vi "Button Appearance Properties.vi"(8 "Error In":errorcluster, 9 "Bool Refnum":refnum<vi>, 11 "Display State In":T1 caption="State") -> (0 "Error Out":errorcluster, 3 "Display State Out":T1 caption="State", 4 "Change":bool)   [LabVIEW 2012, in "Hover Button.xctl"]
doc: "This vi is the interactive property page used to define the color and text properties of the Hover Button."
uses:
  Hover Button.xctl
  State.ctl
  Button Colors.ctl
  Font Properties.ctl
  Color Select.ctl
  <vilib>/Utility/miscctls.llb/LVBoundsTypeDef.ctl
panel:
  in  "Tab Control":enum32{"Appearance", "Font"}(tab)
  in  "On":u32(colorbox)=16860
  in  "Text Color":u32(colorbox)=16448250
  in  "Hover On":u32(colorbox)=16776960
  in  "Hover Text Color":u32(colorbox)
  in  "Example Button":bool
  in  "On text":string
  in  "Off Text":string="Off"
  in  "Off":u32(colorbox)=16860
  in  "Hover Off":u32(colorbox)=16776960
  in  "Show Boolean Text":bool
  in  "Mulitiple strings":bool
  in  "Size":u32=1 min=1 step=1
  in  "Strikeout":bool
  in  "Underline":bool
  in  "Italic":bool
  in  "Bold":bool
  in  "Plain":bool
  out "Example String":string="The quick brown fox jumped over the lazy dog"
  in  "Font":u16(ring) items=["App Font", "Sys Font", "Dlg Font", "ADMUI3.fon", "Agency FB", "Agency FB Bold", "Arial", "Arial Baltic", "Arial Black", "Arial Bold", "Arial Bold Italic", "Arial CE", "Arial CYR", "Arial Greek", "Arial Italic", "Arial Narrow", "Arial Narrow Bold", "Arial Narrow Bold Italic", "Arial Narrow Italic", "Arial Rounded MT Bold", "Arial TUR", "Arial Unicode MS", "Blackadder ITC", "Bodoni MT", "Bodoni MT Black", "Bodoni MT Black Italic", "Bodoni MT Bold", "Bodoni MT Bold Italic", "Bodoni MT Condensed", "Bodoni MT Condensed Bold", "Bodoni MT Condensed Bold Italic", "Bodoni MT Condensed Italic", "Bodoni MT Italic", "Book Antiqua", "Book Antiqua Bold", "Book Antiqua Bold Italic", "Book Antiqua Italic", "Bookman Old Style", "Bookman Old Style Bold", "Bookman Old Style Bold Italic", "Bookman Old Style Italic", "Bookshelf Symbol 7", "Bradley Hand ITC", "Calibri", "Calibri Bold", "Calibri Bold Italic", "Calibri Italic", "Calisto MT", "Calisto MT Bold", "Calisto MT Bold Italic", "Calisto MT Italic", "Cambria & Cambria Math", "Cambria Bold", "Cambria Bold Italic", "Cambria Italic", "Candara", "Candara Bold", "Candara Bold Italic", "Candara Italic", "Castellar", "Century Gothic", "Century Gothic Bold", "Century Gothic Bold Italic", "Century Gothic Italic", "Century Schoolbook", "Century Schoolbook Bold", "Century Schoolbook Bold Italic", "Century Schoolbook Italic", "Comic Sans MS", "Comic Sans MS Bold", "Consolas", "Consolas Bold", "Consolas Bold Italic", "Consolas Italic", "Constantia", "Constantia Bold", "Constantia Bold Italic", "Constantia Italic", "Copperplate Gothic Bold", "Copperplate Gothic Light", "Corbel", "Corbel Bold", "Corbel Bold Italic", "Corbel Italic", "Courier 10,12,15", "Courier New", "Courier New Baltic", "Courier New Bold", "Courier New Bold Italic", "Courier New CE", "Courier New CYR", "Courier New Greek", "Courier New Italic", "Courier New TUR", "Curlz MT", "Edwardian Script ITC", "Elephant", "Elephant Italic", "Engravers MT", "Eras Bold ITC", "Eras Demi ITC", "Eras Light ITC", "Eras Medium ITC", "Estrangelo Edessa", "Estrangelo Edessa", "Euro Sign", "Felix Titling", "Forte", "Franklin Gothic Book", "Franklin Gothic Book Italic", "Franklin Gothic Demi", "Franklin Gothic Demi Cond", "Franklin Gothic Demi Italic", "Franklin Gothic Heavy", "Franklin Gothic Heavy Italic", "Franklin Gothic Medium", "Franklin Gothic Medium Cond", "Franklin Gothic Medium Italic", "French Script MT", "Garamond", "Garamond Bold", "Garamond Italic", "Gautami", "Georgia", "Georgia Bold", "Georgia Bold Italic", "Georgia Italic", "Gigi", "Gill Sans MT", "Gill Sans MT Bold", "Gill Sans MT Bold Italic", "Gill Sans MT Condensed", "Gill Sans MT Ext Condensed Bold", "Gill Sans MT Italic", "Gill Sans Ultra Bold", "Gill Sans Ultra Bold Condensed", "Gloucester MT Extra Condensed", "Goudy Old Style", "Goudy Old Style Bold", "Goudy Old Style Italic", "Goudy Stout", "HE_TERMINAL", "Haettenschweiler", "Helv", "Helvetica", "Impact", "Imprint MT Shadow", "Latha", "Lucida Console", "Lucida Sans Demibold Italic", "Lucida Sans Demibold Roman", "Lucida Sans Italic", "Lucida Sans Regular", "Lucida Sans Typewriter Bold", "Lucida Sans Typewriter Bold Oblique", "Lucida Sans Typewriter Oblique", "Lucida Sans Typewriter Regular", "Lucida Sans Unicode", "MS Outlook", "MS Reference Sans Serif", "MS Reference Specialty", "MS Sans Serif 8,10,12,14,18,24", "MS Serif 8,10,12,14,18,24", "MS Shell Dlg", "MS Shell Dlg 2", "MT Extra", "Maiandra GD", "Mangal", "Microsoft Sans Serif", "Modern", "Monotype Corsiva", "Mv Boli", "OCR A Extended", "Palace Script MT", "Palatino Linotype", "Palatino Linotype Bold", "Palatino Linotype Bold Italic", "Palatino Linotype Italic", "Papyrus", "Perpetua", "Perpetua Bold", "Perpetua Bold Italic", "Perpetua Italic", "Perpetua Titling MT Bold", "Perpetua Titling MT Light", "Pristina", "Raavi", "Rage Italic", "Rockwell", "Rockwell Bold", "Rockwell Bold Italic", "Rockwell Condensed", "Rockwell Condensed Bold", "Rockwell Extra Bold", "Rockwell Italic", "Roman", "Script", "Script MT Bold", "Shruti", "Small Fonts", "Sylfaen", "Symbol", "Symbol 8,10,12,14,18,24", "Tahoma", "Tahoma Bold", "Times", "Times New Roman", "Times New Roman Baltic", "Times New Roman Bold", "Times New Roman Bold Italic", "Times New Roman CE", "Times New Roman CYR", "Times New Roman Greek", "Times New Roman Italic", "Times New Roman TUR", "Tms Rmn", "Trebuchet MS", "Trebuchet MS Bold", "Trebuchet MS Bold Italic", "Trebuchet MS Italic", "Tunga", "Tw Cen MT", "Tw Cen MT Bold", "Tw Cen MT Bold Italic", "Tw Cen MT Condensed", "Tw Cen MT Condensed Bold", "Tw Cen MT Condensed Extra Bold", "Tw Cen MT Italic", "Verdana", "Verdana Bold", "Verdana Bold Italic", "Verdana Italic", "WST_Czec", "WST_Engl", "WST_Fren", "WST_Germ", "WST_Ital", "WST_Span", "WST_Swed", "Webdings", "WingDings", "Wingdings 2", "Wingdings 3", "ZWAdobeF"]
  in  "Alignment":enum16{"Left", "Center", "Right"}(ring)
  in  "Cancel Button":bool
  in  "OK Button":bool
  # "Appearance"
  # "Colors"
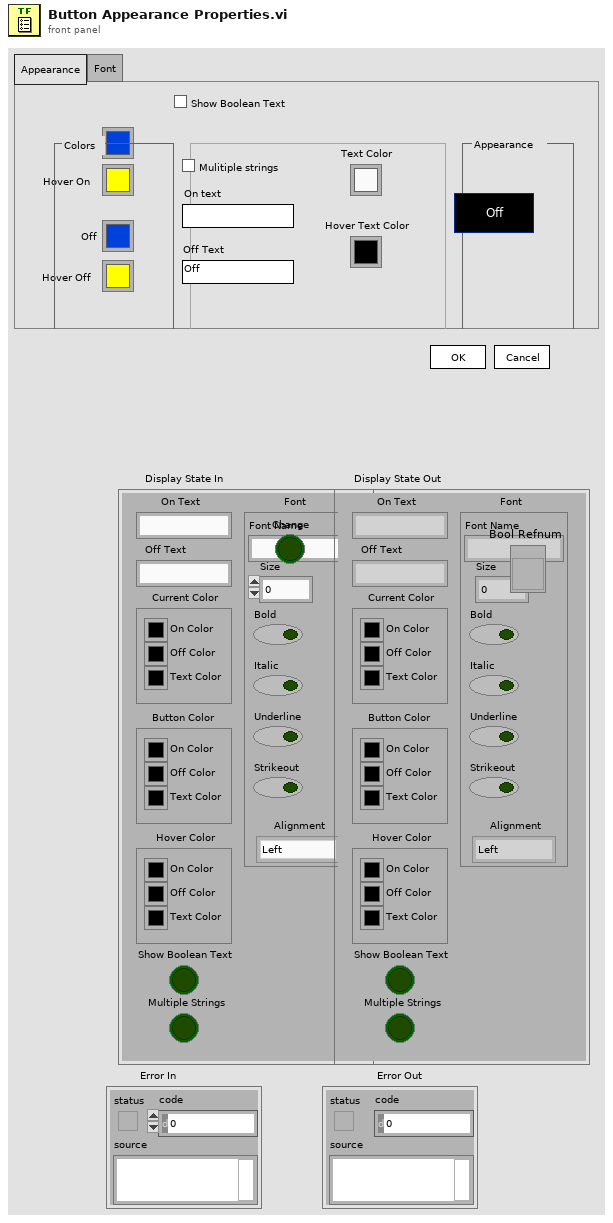
[diagram p1: front panel]
types:
  T1 = typedef "Hover Button.xctl/State.ctl" = cluster{"On Text":string, "Off Text":string, "Current Color":T2, "Button Color":T2, "Hover Color":T2, "Show Boolean Text":bool, "Multiple Strings":bool, "Font":T3}
  T2 = typedef "Hover Button.xctl/Button Colors.ctl" = cluster{"On Color":u32, "Text Color":u32, "Off Color":u32}
  T3 = typedef "Hover Button.xctl/Font Properties.ctl" = cluster{"Font Name":string, "Size":u32, "Bold":bool, "Italic":bool, "Underline":bool, "Strikeout":bool, "Alignment":enum16{"Left", "Center", "Right"}}
  T4 = typedef "Hover Button.xctl/Color Select.ctl" = enum16{"Current Color", "Button Color", "Hover Color"}
  T5 = typedef "LVBoundsTypeDef.ctl" = cluster{"Width":u32, "Height":u32}
  T6 = cluster{"Text Color":u32, "Background Color":u32}
  T7 = typedef "LVPositionTypeDef.ctl" = cluster{"Left":i32, "Top":i32}
  T8 = cluster{"On Text":bool, "Off Text":bool, "Current Color":cluster{"On Color":bool, "Text Color":bool, "Off Color":bool}, "Button Color":cluster{"On Color":bool, "Text Color":bool, "Off Color":bool}, "Hover Color":cluster{"On Color":bool, "Text Color":bool, "Off Color":bool}, "Show Boolean Text":bool, "Multiple Strings":bool, "Font":cluster{"Font Name":bool, "Size":bool, "Bold":bool, "Italic":bool, "Underline":bool, "Strikeout":bool, "Alignment":bool}}
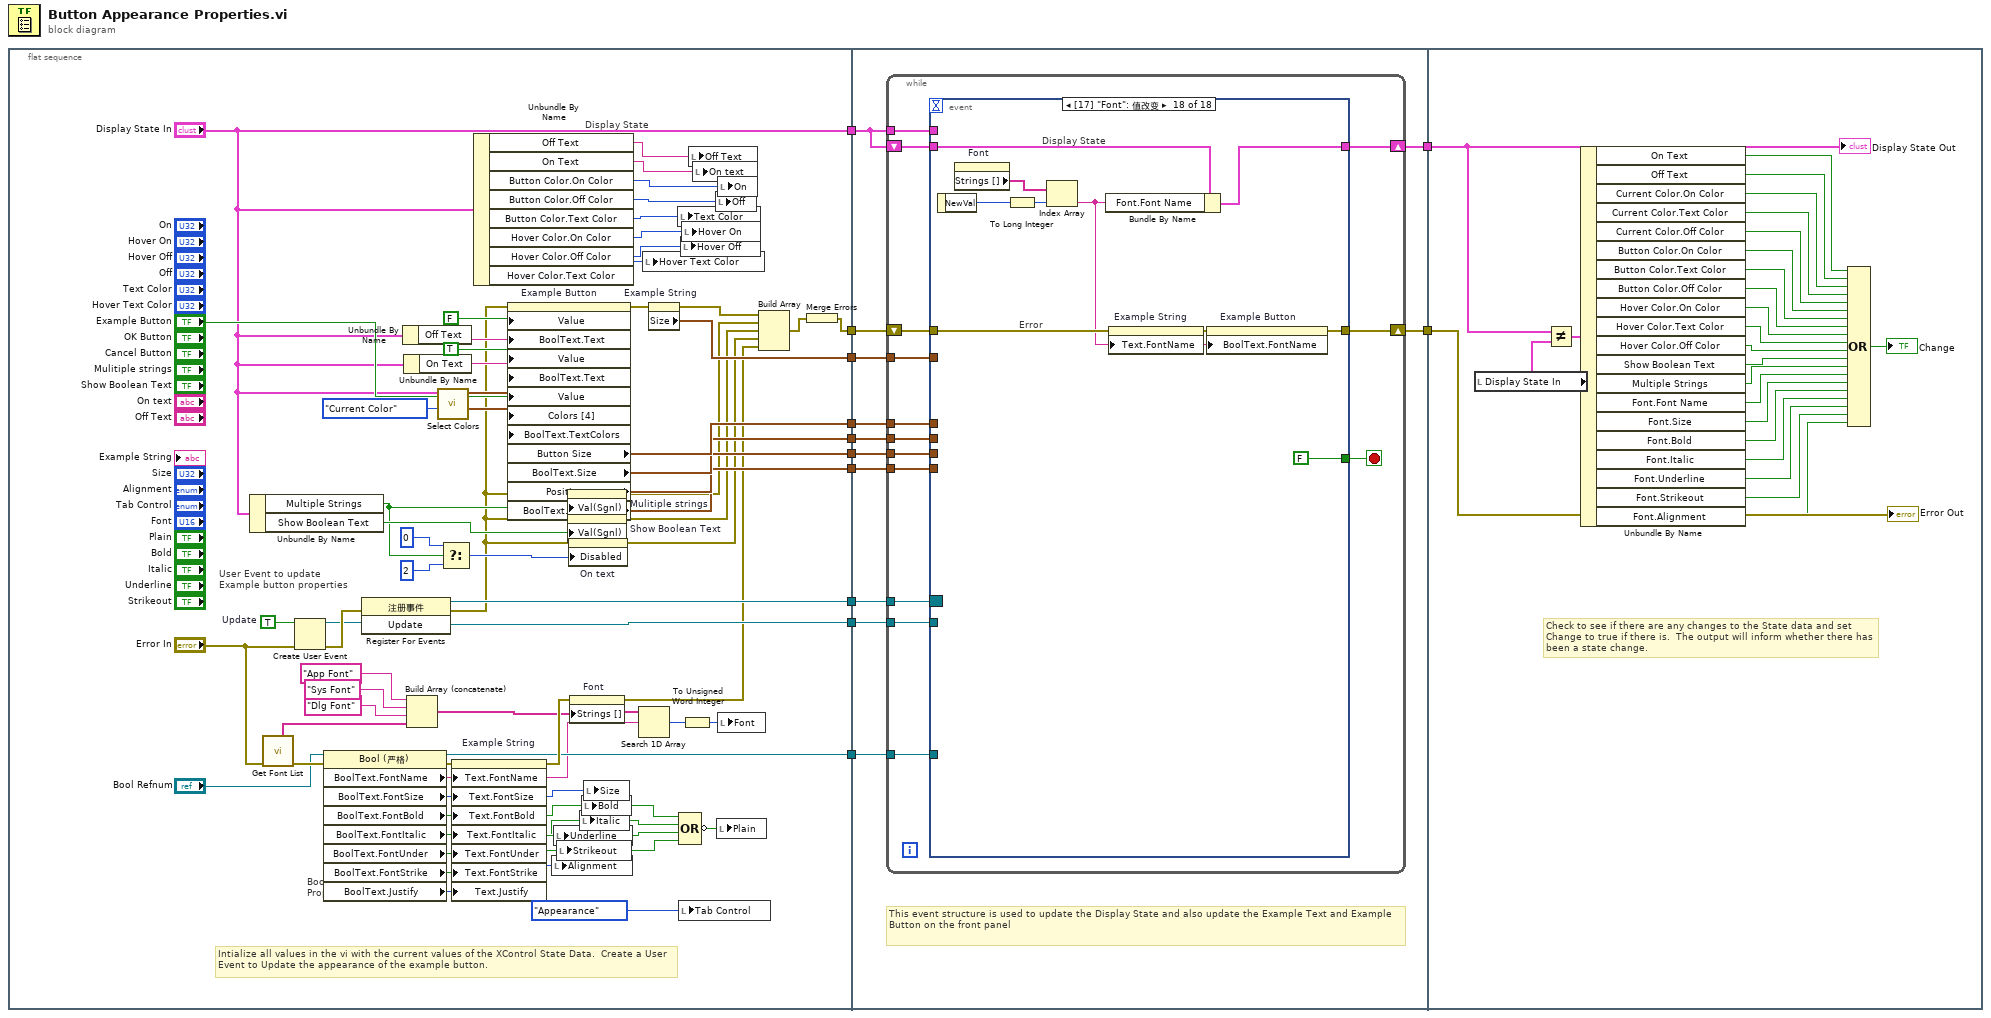
[diagram p0: block diagram]
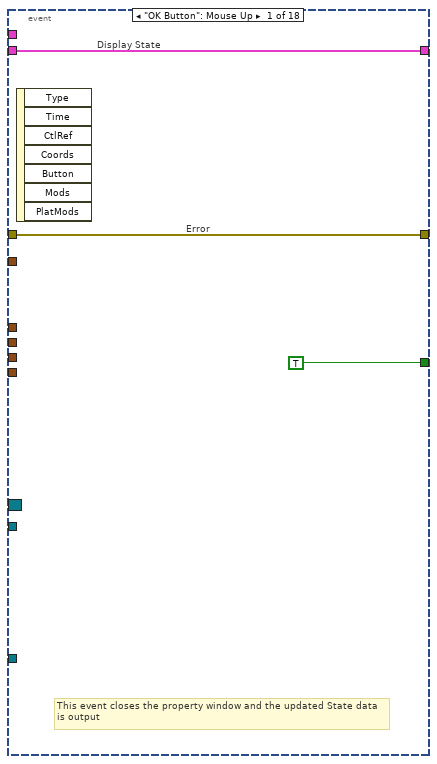
[diagram p2: hidden frame]
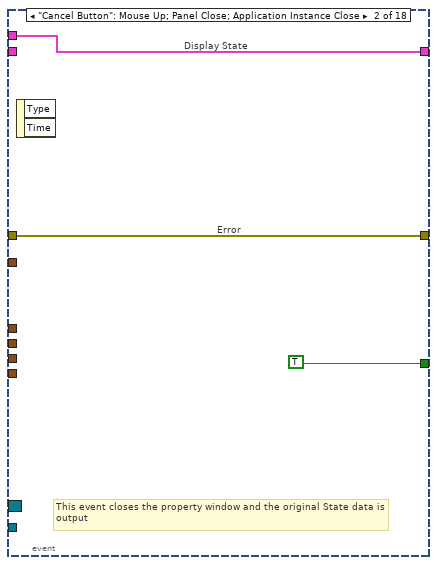
[diagram p3: hidden frame]
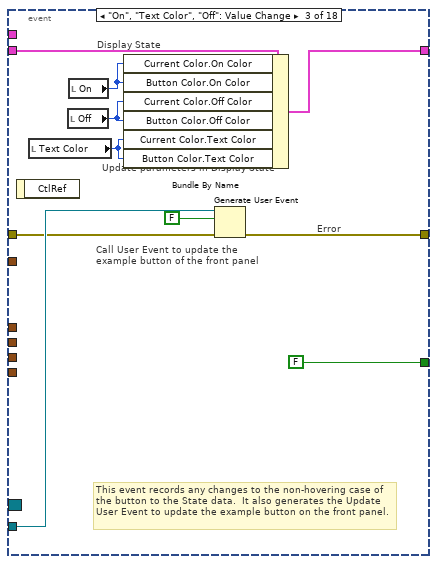
[diagram p4: hidden frame]
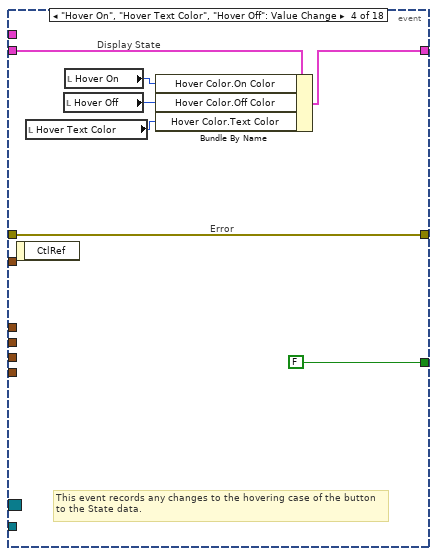
[diagram p5: hidden frame]
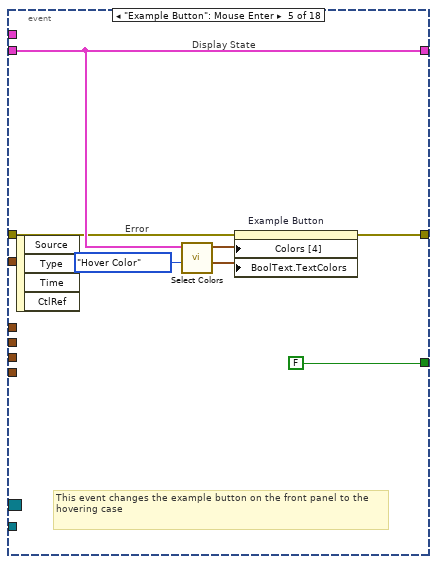
[diagram p6: hidden frame]
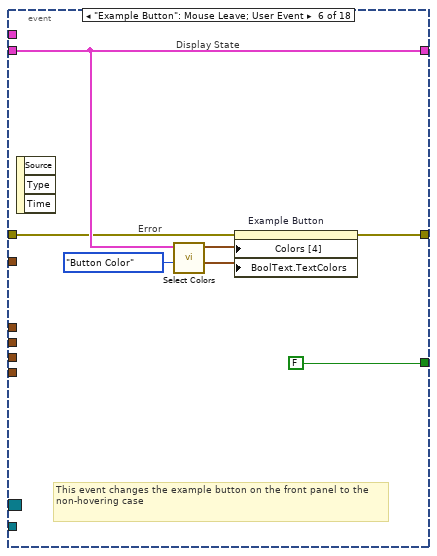
[diagram p7: hidden frame]
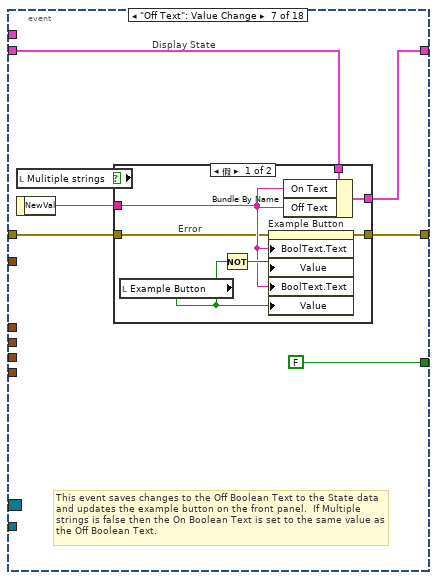
[diagram p8: hidden frame]
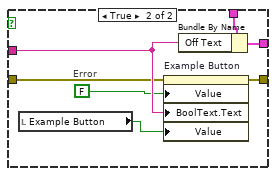
[diagram p9: hidden frame]
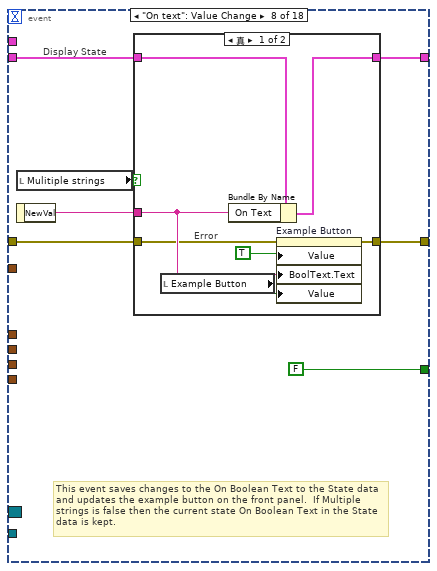
[diagram p10: hidden frame]
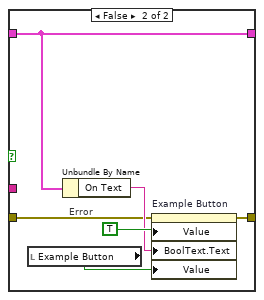
[diagram p11: hidden frame]
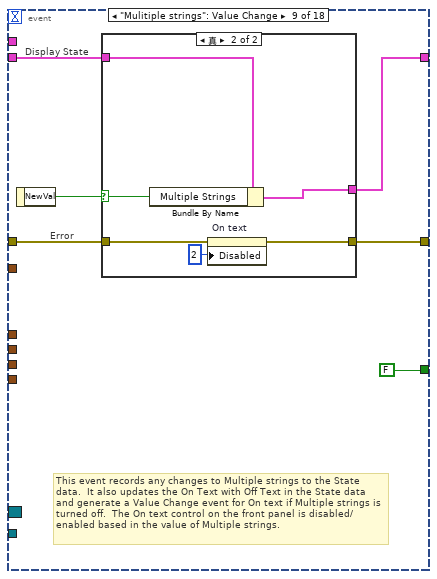
[diagram p12: hidden frame]
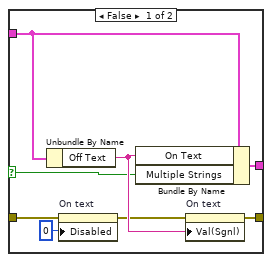
[diagram p13: hidden frame]
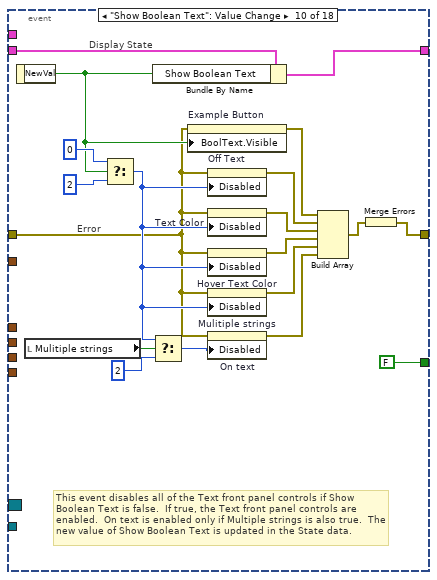
[diagram p14: hidden frame]
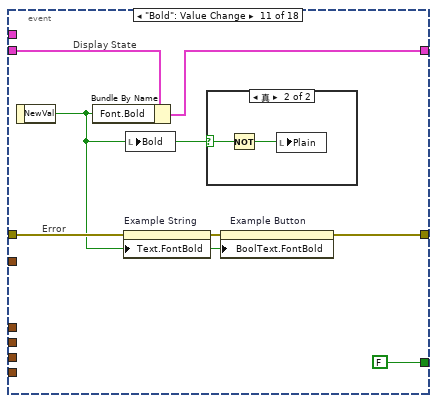
[diagram p15: hidden frame]
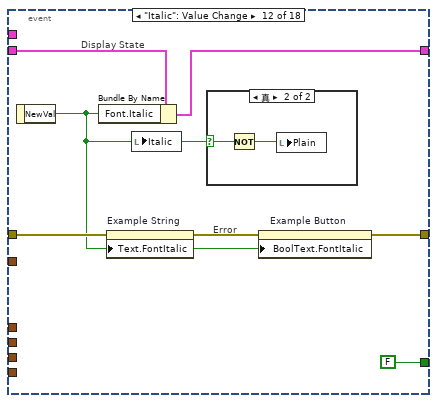
[diagram p17: hidden frame]
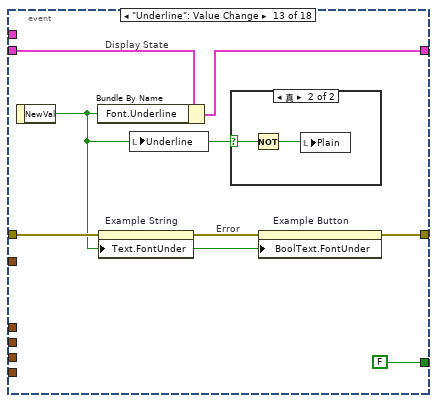
[diagram p19: hidden frame]
diagram:
  n1 = flat-sequence {
    tunnel: ["Display State In"] -> w12
    tunnel: [w26] -> w10
    tunnel: [w25] -> w9
    tunnel: [w54] -> w8
    tunnel: [w47] -> w6
    tunnel: [w27] -> w5
    tunnel: [w33] -> w4
    tunnel: [w32] -> w3
    tunnel: [w31] -> w2
    tunnel: [w30] -> w1
    tunnel: w12 -> [w86]
    tunnel: [w85] -> w11
    tunnel: w10 -> [w84]
    tunnel: w9 -> [w83]
    tunnel: w8 -> [w82]
    tunnel: [w81] -> w7
    tunnel: w6 -> [w80]
    tunnel: w5 -> [w79]
    tunnel: w4 -> [w78]
    tunnel: w3 -> [w77]
    tunnel: w2 -> [w76]
    tunnel: w1 -> [w75]
    tunnel: w11 -> [w317]
    tunnel: w7 -> [w302]
    frame #0 {
      w72 = TRUE  # Update
      # "User Event to update\nExample button properties"
      # "Boolean Button Reference\nProperties"
      # "Display State"
      # "Intialize all values in the vi with the current values of the XControl State Data.  Create a User Event to Update the appearance of the example button."
      n2 = Unbundle By Name("Display State In") -> ("Multiple Strings"=w55:bool, "Show Boolean Text"=w58:bool)
      n3 = call "Get Font List.vi"("Error In"="Error In") -> ("Error Out"=w74:errorcluster, "Font Array"=w28:string[])  [unwired: 9 in]
      n4 = Create User Event(user event datatype=w72, error in="Error In") -> (user event=w25:refnum<user-event>, error out=w35:errorcluster)
      n5 = property class="Bool (严格)"(reference="Bool Refnum", error in=w74) -> (reference out=w47:refnum<vi>, error out=w36:errorcluster, "BoolText.FontName"=w37:string, "BoolText.FontSize"=w38:u32, "BoolText.FontBold"=w39:bool, "BoolText.FontItalic"=w40:bool, "BoolText.FontUnder"=w41:bool, "BoolText.FontStrike"=w42:bool, "BoolText.Justify"=w43:enum16{"Left", "Center", "Right"})
      n6 = register-events(error in=w35, w25) -> (reference out=w26:refnum<event-registration>, error out=w19:errorcluster)  [unwired: 1 in]
      n7 = Unbundle By Name("Display State In") -> ("Off Text"=w67:string)
      n8 = Unbundle By Name("Display State In") -> ("On Text"=w66:string)
      n9 = Build Array (concatenate)("App Font", "Sys Font", "Dlg Font", w28) -> (w50:string[])
      n10 = call "Select Colors.vi"("Color Select"=Color_Select."Current Color", "State"="Display State In") -> ("Text Colors"=w56:T6, "Button Colors"=w57:cluster{"FG":u32, "BG":u32}[])  [unwired: 8 in]
      n11 = Select(t=u8 0, s=w55, f=u8 2) -> (s? t:f=w59:u8)
      n12 = property on="Example String" class="Str"(error in=w36, "Text.FontName"=w37, "Text.FontSize"=w38, "Text.FontBold"=w39, "Text.FontItalic"=w40, "Text.FontUnder"=w41, "Text.FontStrike"=w42, "Text.Justify"=w43) -> (error out=w73:errorcluster)  [unwired: 1 in, 1 out]
      n13 = Unbundle By Name("Display State In") -> ("Off Text"=w20:string, "On Text"=w21:string, "Button Color.On Color"=w22:u32, "Button Color.Off Color"=w23:u32, "Button Color.Text Color"=w24:u32, "Hover Color.On Color"=w70:u32, "Hover Color.Off Color"=w69:u32, "Hover Color.Text Color"=w68:u32)
      n14 = property on="Example Button" class="Bool (严格)"(error in=w19, "Value"=FALSE ("Boolean"), "BoolText.Text"=w67, "Value"=TRUE ("Boolean"), "BoolText.Text"=w66, "Value"="Example Button", "Colors [4]"=w57, "BoolText.TextColors"=w56) -> (error out=w29:errorcluster, "Button Size"=w33:T5, "BoolText.Size"=w32:T5, "Position"=w31:T7, "BoolText.Position"=w30:T7)  [unwired: 1 in, 1 out]
      n15 = local write "Alignment"(w43) -> ()
      n16 = local write "Underline"(w41) -> ()
      n17 = local write "Strikeout"(w42) -> ()
      n18 = property on="Mulitiple strings" class="Bool (严格)"(error in=w19, "Val(Sgnl)"=w55) -> (error out=w15:errorcluster)  [unwired: 1 in, 1 out]
      n19 = property on="Show Boolean Text" class="Bool (严格)"(error in=w19, "Val(Sgnl)"=w58) -> (error out=w16:errorcluster)  [unwired: 1 in, 1 out]
      n20 = property on="On text" class="Str"(error in=w19, "Disabled"=w59) -> (error out=w17:errorcluster)  [unwired: 1 in, 1 out]
      n21 = property on="Font" class="Ring (严格)"(error in=w73, "Strings []"=w50) -> (error out=w18:errorcluster)  [unwired: 1 in, 1 out]
      n22 = local write "Italic"(w40) -> ()
      n23 = local write "Bold"(w39) -> ()
      n24 = local write "Size"(w38) -> ()
      n25 = Search 1D Array(1D array=w50, element=w37) -> (index of element=w48:i32)  [unwired: 1 in]
      n26 = local write "Hover Text Color"(w68) -> ()
      n27 = property on="Example String" class="Str"(error in=w29) -> (error out=w14:errorcluster, "Size"=w27:T5)  [unwired: 1 in, 1 out]
      n28 = local write "Text Color"(w24) -> ()
      n29 = Compound Arithmetic op=OR(w39, w40, w41, w42) -> (invert w45:bool)
      n30 = local write "Tab Control"(enum32{"Appearance", "Font"}."Appearance" ("Tab Control")) -> ()
      n31 = local write "Hover Off"(w69) -> ()
      n32 = local write "Hover On"(w70) -> ()
      n33 = To Unsigned Word Integer(number=w48) -> (unsigned 16bit integer=w46:u16)
      n34 = local write "Off Text"(w20) -> ()
      n35 = local write "On text"(w21) -> ()
      n36 = local write "Off"(w23) -> ()
      n37 = local write "Plain"(w45) -> ()
      n38 = local write "On"(w22) -> ()
      n39 = local write "Font"(w46) -> ()
      n40 = Build Array(w14, w15, w16, w17, w18) -> (w13:errorcluster[])
      n41 = Merge Errors(w13) -> (w54:errorcluster)
    }
    frame #1 {
      # "This event structure is used to update the Display State and also update the Example Text and Example Button on the front panel"
      n42 = while {
        tunnel: w86 -> [w97]
        shift-right: [w98] -> w85
        shift-left: w86 -> [w99]
        tunnel: w84 -> [w96]
        tunnel: w83 -> [w95]
        shift-right: [w93] -> w81
        shift-left: w82 -> [w94]
        tunnel: w80 -> [w92]
        tunnel: w79 -> [w91]
        tunnel: w78 -> [w90]
        tunnel: w77 -> [w89]
        tunnel: w76 -> [w88]
        tunnel: w75 -> [w87]
        stop <- w100 stop-if-true
        n43 = event shown="[17] \"Font\": 值改变" {
          selector: w96 -> [_ _ _ _ _ _ _ _ _ _ _ _ _ _ _ _ _ _]
          dyn-events: _ -> [_ _ _ _ _ _ _ _ _ _ _ _ _ _ _ _ _ _]
          timeout: _ -> [_ _ _ _ _ _ _ _ _ _ _ _ _ _ _ _ _ _]
          tunnel: [TRUE TRUE FALSE FALSE FALSE FALSE FALSE FALSE FALSE FALSE FALSE FALSE FALSE FALSE FALSE FALSE FALSE FALSE] -> w100
          tunnel: w99 -> [w102 _ w116 w123 w129 w133 w144 w165 w182 w216 w224 w233 w242 w251 w260 w275 w282 w292]
          tunnel: [w102 w105 w114 w121 w129 w133 w143 w164 w181 w215 w223 w232 w241 w250 w259 w274 w281 w291] -> w98
          tunnel: w97 -> [_ w105 _ _ _ _ _ _ _ _ _ _ _ _ _ _ _ _]
          tunnel: w95 -> [_ _ w112 _ _ _ _ _ _ _ _ _ _ _ _ _ _ _]
          tunnel: w94 -> [w101 w104 w108 w117 w125 w132 w138 w159 w180 w200 w221 w230 w239 w248 w257 w262 w280 w287]
          tunnel: [w101 w104 w107 w117 w124 w131 w139 w160 w179 w207 w219 w228 w236 w245 w254 w271 w278 w285] -> w93
          tunnel: w92 -> [_ _ _ _ _ _ _ _ _ _ _ _ _ _ _ _ _ _]
          tunnel: w91 -> [_ _ _ _ _ _ _ _ _ _ _ _ _ _ _ w273 _ _]
          tunnel: w90 -> [_ _ _ _ _ _ _ _ _ _ _ _ _ _ _ w268 _ _]
          tunnel: w89 -> [_ _ _ _ _ _ _ _ _ _ _ _ _ _ _ _ _ _]
          tunnel: w88 -> [_ _ _ _ _ _ _ _ _ _ _ _ _ _ _ w264 _ _]
          tunnel: w87 -> [_ _ _ _ _ _ _ _ _ _ _ _ _ _ _ _ _ _]
          event "OK Button": Mouse Up {
            # "Error"
            # "Display State"
            # "This event closes the property window and the updated State data is output"
            n44 = event-data() -> ()  [unwired: 1 in, 7 out]
          }
          event "Cancel Button": Mouse Up; Panel Close; Application Instance Close {
            # "Error"
            # "Display State"
            # "This event closes the property window and the original State data is output"
            n45 = event-data() -> ()  [unwired: 1 in, 2 out]
          }
          event "On", "Text Color", "Off": Value Change {
            # "Error"
            # "Display State"
            # "Update parameters in Display State"
            # "Call User Event to update the\nexample button of the front panel"
            # "This event records any changes to the non-hovering case of the button to the State data.  It also generates the Update User Event to update the example button on the front panel."
            n46 = event-data() -> ()  [unwired: 1 in, 1 out]
            n47 = local read "Text Color"() -> (w115:u32)
            n48 = local read "Off"() -> (w109:u32)
            n49 = local read "On"() -> (w110:u32)
            n50 = Bundle By Name(cluster=w116, "Current Color.On Color"=w110, "Button Color.On Color"=w110, "Current Color.Off Color"=w109, "Button Color.Off Color"=w109, "Current Color.Text Color"=w115, "Button Color.Text Color"=w115) -> (w114:T1)
            n51 = Generate User Event(user event=w112, event data cluster=FALSE ("event data"), error in=w108) -> (error out=w107:errorcluster)  [unwired: 1 out]
          }
          event "Hover On", "Hover Text Color", "Hover Off": Value Change {
            # "Error"
            # "Display State"
            # "This event records any changes to the hovering case of the button to the State data."
            n52 = event-data() -> ()  [unwired: 1 in, 1 out]
            n53 = local read "Hover Text Color"() -> (w122:u32)
            n54 = local read "Hover Off"() -> (w119:u32)
            n55 = local read "Hover On"() -> (w118:u32)
            n56 = Bundle By Name(cluster=w123, "Hover Color.On Color"=w118, "Hover Color.Off Color"=w119, "Hover Color.Text Color"=w122) -> (w121:T1)
          }
          event "Example Button": Mouse Enter {
            # "Error"
            # "Display State"
            # "This event changes the example button on the front panel to the hovering case"
            n57 = event-data() -> ()  [unwired: 1 in, 4 out]
            n58 = call "Select Colors.vi"("Color Select"=Color_Select."Hover Color", "State"=w129) -> ("Text Colors"=w127:T6, "Button Colors"=w128:cluster{"FG":u32, "BG":u32}[])  [unwired: 8 in]
            n59 = property on="Example Button" class="Bool (严格)"(error in=w125, "Colors [4]"=w128, "BoolText.TextColors"=w127) -> (error out=w124:errorcluster)  [unwired: 1 in, 1 out]
          }
          event "Example Button": Mouse Leave; User Event {
            # "Error"
            # "Display State"
            # "This event changes the example button on the front panel to the non-hovering case"
            n60 = event-data() -> ()  [unwired: 1 in, 3 out]
            n61 = call "Select Colors.vi"("Color Select"=Color_Select."Button Color", "State"=w133) -> ("Text Colors"=w135:T6, "Button Colors"=w136:cluster{"FG":u32, "BG":u32}[])  [unwired: 8 in]
            n62 = property on="Example Button" class="Bool (严格)"(error in=w132, "Colors [4]"=w136, "BoolText.TextColors"=w135) -> (error out=w131:errorcluster)  [unwired: 1 in, 1 out]
          }
          event "Off Text": Value Change {
            # "Display State"
            # "This event saves changes to the Off Boolean Text to the State data and updates the example button on the front panel.  If Multiple strings is false then the On Boolean Text is set to the same value as the Off Boolean Text."
            n63 = local read "Mulitiple strings"() -> (w140:bool)
            n64 = event-data() -> ("NewVal"=w141:string)  [unwired: 1 in]
            n65 = case shown="假" w140 {
              tunnel: w144 -> [w151 w158]
              tunnel: [w150 w157] -> w143
              tunnel: w141 -> [w147 w155]
              tunnel: [w146 w153] -> w139
              tunnel: w138 -> [w145 w152]
              frame False {
                # "Error"
                n66 = local read "Example Button"() -> (w149:bool)
                n67 = Not(x=w149) -> (.not. x?=w148:bool)
                n68 = property on="Example Button" class="Bool (严格)"(error in=w145, "BoolText.Text"=w147, "Value"=w148, "BoolText.Text"=w147, "Value"=w149) -> (error out=w146:errorcluster)  [unwired: 1 in, 1 out]
                n69 = Bundle By Name(cluster=w151, "On Text"=w147, "Off Text"=w147) -> (w150:T1)
              }
              frame True {
                # "Error"
                n70 = local read "Example Button"() -> (w156:bool)
                n71 = property on="Example Button" class="Bool (严格)"(error in=w152, "Value"=FALSE ("Boolean"), "BoolText.Text"=w155, "Value"=w156) -> (error out=w153:errorcluster)  [unwired: 1 in, 1 out]
                n72 = Bundle By Name(cluster=w158, "Off Text"=w155) -> (w157:T1)
              }
            }
          }
          event "On text": Value Change {
            # "Display State"
            # "This event saves changes to the On Boolean Text to the State data and updates the example button on the front panel.  If Multiple strings is false then the current state On Boolean Text in the State data is kept."
            n73 = local read "Mulitiple strings"() -> (w162:bool)
            n74 = event-data() -> ("NewVal"=w161:string)  [unwired: 1 in]
            n75 = case shown="真" w162 {
              tunnel: w165 -> [w172 w176]
              tunnel: [w171 w176] -> w164
              tunnel: w161 -> [w169 _]
              tunnel: [w167 w174] -> w160
              tunnel: w159 -> [w166 w173]
              frame True {
                # "Error"
                n76 = local read "Example Button"() -> (w170:bool)
                n77 = Bundle By Name(cluster=w172, "On Text"=w169) -> (w171:T1)
                n78 = property on="Example Button" class="Bool (严格)"(error in=w166, "Value"=TRUE ("Boolean"), "BoolText.Text"=w169, "Value"=w170) -> (error out=w167:errorcluster)  [unwired: 1 in, 1 out]
              }
              frame False {
                # "Error"
                n79 = local read "Example Button"() -> (w178:bool)
                n80 = Unbundle By Name(w176) -> ("On Text"=w175:string)
                n81 = property on="Example Button" class="Bool (严格)"(error in=w173, "Value"=TRUE ("Boolean"), "BoolText.Text"=w175, "Value"=w178) -> (error out=w174:errorcluster)  [unwired: 1 in, 1 out]
              }
            }
          }
          event "Mulitiple strings": Value Change {
            # "Error"
            # "Display State"
            # "This event records any changes to Multiple strings to the State data.  It also updates the On Text with Off Text in the State data and generate a Value Change event for On text if Multiple strings is turned off.  The On text control on the front panel is disabled/enabled based in the value of Multiple strings."
            n82 = event-data() -> ("NewVal"=w183:bool)  [unwired: 1 in]
            n83 = case shown="真" w183 {
              selector: w183 -> [w190 w198]
              tunnel: w182 -> [w192 w197]
              tunnel: [w189 w196] -> w181
              tunnel: w180 -> [w186 w195]
              tunnel: [w185 w194] -> w179
              frame False {
                n84 = Unbundle By Name(w192) -> ("Off Text"=w191:string)
                n85 = property on="On text" class="Str"(error in=w186, "Disabled"=u8 0) -> (error out=w188:errorcluster)  [unwired: 1 in, 1 out]
                n86 = Bundle By Name(cluster=w192, "On Text"=w191, "Multiple Strings"=w190) -> (w189:T1)
                n87 = property on="On text" class="Str"(error in=w188, "Val(Sgnl)"=w191) -> (error out=w185:errorcluster)  [unwired: 1 in, 1 out]
              }
              frame True {
                n88 = Bundle By Name(cluster=w197, "Multiple Strings"=w198) -> (w196:T1)
                n89 = property on="On text" class="Str"(error in=w195, "Disabled"=u8 2) -> (error out=w194:errorcluster)  [unwired: 1 in, 1 out]
              }
            }
          }
          event "Show Boolean Text": Value Change {
            # "Error"
            # "Display State"
            # "This event disables all of the Text front panel controls if Show Boolean Text is false.  If true, the Text front panel controls are enabled.  On text is enabled only if Multiple strings is also true.  The new value of Show Boolean Text is updated in the State data."
            n90 = event-data() -> ("NewVal"=w212:bool)  [unwired: 1 in]
            n91 = local read "Mulitiple strings"() -> (w211:bool)
            n92 = Select(t=u8 0, s=w212, f=u8 2) -> (s? t:f=w210:u8)
            n93 = Bundle By Name(cluster=w216, "Show Boolean Text"=w212) -> (w215:T1)
            n94 = Select(t=w210, s=w211, f=u8 2) -> (s? t:f=w209:u8)
            n95 = property on="Example Button" class="Bool (严格)"(error in=w200, "BoolText.Visible"=w212) -> (error out=w199:errorcluster)  [unwired: 1 in, 1 out]
            n96 = property on="Off Text" class="Str"(error in=w200, "Disabled"=w210) -> (error out=w204:errorcluster)  [unwired: 1 in, 1 out]
            n97 = property on="Text Color" class="ColBox"(error in=w200, "Disabled"=w210) -> (error out=w205:errorcluster)  [unwired: 1 in, 1 out]
            n98 = property on="Hover Text Color" class="ColBox"(error in=w200, "Disabled"=w210) -> (error out=w206:errorcluster)  [unwired: 1 in, 1 out]
            n99 = property on="Mulitiple strings" class="Bool (严格)"(error in=w200, "Disabled"=w210) -> (error out=w203:errorcluster)  [unwired: 1 in, 1 out]
            n100 = property on="On text" class="Str"(error in=w200, "Disabled"=w209) -> (error out=w202:errorcluster)  [unwired: 1 in, 1 out]
            n101 = Build Array(w199, w204, w205, w206, w203, w202) -> (w201:errorcluster[])
            n102 = Merge Errors(w201) -> (w207:errorcluster)
          }
          event "Bold": Value Change {
            # "Error"
            # "Display State"
            n103 = event-data() -> ("NewVal"=w218:bool)  [unwired: 1 in]
            n104 = Bundle By Name(cluster=w224, "Font.Bold"=w218) -> (w223:T1)
            n105 = property on="Example String" class="Str"(error in=w221, "Text.FontBold"=w218) -> (error out=w220:errorcluster)  [unwired: 1 in, 1 out]
            n106 = local write "Bold"(w218) -> ()
            n107 = case shown="真" w218 {
              selector: w218 -> [_ w226]
              frame False {
              }
              frame True {
                n108 = Not(x=w226) -> (.not. x?=w225:bool)
                n109 = local write "Plain"(w225) -> ()
              }
            }
            n110 = property on="Example Button" class="Bool (严格)"(error in=w220, "BoolText.FontBold"=w218) -> (error out=w219:errorcluster)  [unwired: 1 in, 1 out]
          }
          event "Italic": Value Change {
            # "Error"
            # "Display State"
            n111 = event-data() -> ("NewVal"=w227:bool)  [unwired: 1 in]
            n112 = Bundle By Name(cluster=w233, "Font.Italic"=w227) -> (w232:T1)
            n113 = property on="Example String" class="Str"(error in=w230, "Text.FontItalic"=w227) -> (error out=w229:errorcluster)  [unwired: 1 in, 1 out]
            n114 = local write "Italic"(w227) -> ()
            n115 = case shown="真" w227 {
              selector: w227 -> [_ w235]
              frame False {
              }
              frame True {
                n116 = Not(x=w235) -> (.not. x?=w234:bool)
                n117 = local write "Plain"(w234) -> ()
              }
            }
            n118 = property on="Example Button" class="Bool (严格)"(error in=w229, "BoolText.FontItalic"=w227) -> (error out=w228:errorcluster)  [unwired: 1 in, 1 out]
          }
          event "Underline": Value Change {
            # "Error"
            # "Display State"
            n119 = event-data() -> ("NewVal"=w238:bool)  [unwired: 1 in]
            n120 = Bundle By Name(cluster=w242, "Font.Underline"=w238) -> (w241:T1)
            n121 = property on="Example String" class="Str"(error in=w239, "Text.FontUnder"=w238) -> (error out=w237:errorcluster)  [unwired: 1 in, 1 out]
            n122 = local write "Underline"(w238) -> ()
            n123 = case shown="真" w238 {
              selector: w238 -> [_ w244]
              frame False {
              }
              frame True {
                n124 = Not(x=w244) -> (.not. x?=w243:bool)
                n125 = local write "Plain"(w243) -> ()
              }
            }
            n126 = property on="Example Button" class="Bool (严格)"(error in=w237, "BoolText.FontUnder"=w238) -> (error out=w236:errorcluster)  [unwired: 1 in, 1 out]
          }
          event "Strikeout": Value Change {
            # "Error"
            # "Display State"
            n127 = event-data() -> ("NewVal"=w247:bool)  [unwired: 1 in]
            n128 = Bundle By Name(cluster=w251, "Font.Strikeout"=w247) -> (w250:T1)
            n129 = property on="Example String" class="Str"(error in=w248, "Text.FontStrike"=w247) -> (error out=w246:errorcluster)  [unwired: 1 in, 1 out]
            n130 = local write "Strikeout"(w247) -> ()
            n131 = case shown="真" w247 {
              selector: w247 -> [_ w253]
              frame False {
              }
              frame True {
                n132 = Not(x=w253) -> (.not. x?=w252:bool)
                n133 = local write "Plain"(w252) -> ()
              }
            }
            n134 = property on="Example Button" class="Bool (严格)"(error in=w246, "BoolText.FontUnder"=w247) -> (error out=w245:errorcluster)  [unwired: 1 in, 1 out]
          }
          event "Plain": Value Change {
            w256 = FALSE ("Font.Bold")
            # "Error"
            # "Display State"
            n135 = event-data() -> ()  [unwired: 1 in, 1 out]
            n136 = property on="Example String" class="Str"(error in=w257, "Text.FontBold"=w256, "Text.FontItalic"=w256, "Text.FontUnder"=w256, "Text.FontStrike"=w256) -> (error out=w255:errorcluster)  [unwired: 1 in, 1 out]
            n137 = local write "Underline"(w256) -> ()
            n138 = local write "Strikeout"(w256) -> ()
            n139 = local write "Italic"(w256) -> ()
            n140 = local write "Bold"(w256) -> ()
            n141 = property on="Example Button" class="Bool (严格)"(error in=w255, "BoolText.FontBold"=w256, "BoolText.FontItalic"=w256, "BoolText.FontUnder"=w256, "BoolText.FontStrike"=w256) -> (error out=w254:errorcluster)  [unwired: 1 in, 1 out]
            n142 = Bundle By Name(cluster=w260, "Font.Bold"=w256, "Font.Italic"=w256, "Font.Underline"=w256, "Font.Strikeout"=w256) -> (w259:T1)
          }
          event "Size": Value Change {
            # "Error"
            # "Display State"
            n143 = event-data() -> ("NewVal"=w270:u32)  [unwired: 1 in]
            n144 = property on="Example Button" class="Bool (严格)"(error in=w262) -> (error out=w261:errorcluster, "BoolText.Size"=w269:T5)  [unwired: 1 in, 1 out]
            n145 = property on="Example String" class="Str"(error in=w261, "Text.FontSize"=w270, "Size"=w273) -> (error out=w272:errorcluster)  [unwired: 1 in, 1 out]
            n146 = Subtract(x=w268, y=w269) -> (x-y=w267:T5)
            n147 = Bundle By Name(cluster=w275, "Font.Size"=w270) -> (w274:T1)
            n148 = Quotient & Remainder(x=w267, y=T5 {"Width"=2, "Height"=2}) -> (floor(x/y)=w265:T5)  [unwired: 1 out]
            n149 = Add(x=w264, y=w265) -> (x+y=w263:T5)
            n150 = property on="Example Button" class="Bool (严格)"(error in=w272, "BoolText.FontSize"=w270, "Button Size"=w268, "Position"=w264, "BoolText.Position"=w263) -> (error out=w271:errorcluster)  [unwired: 1 in, 1 out]
          }
          event "Alignment": Value Change {
            # "Error"
            # "Display State"
            n151 = event-data() -> ("NewVal"=w277:enum16{"Left", "Center", "Right"})  [unwired: 1 in]
            n152 = Bundle By Name(cluster=w282, "Font.Alignment"=w277) -> (w281:T1)
            n153 = property on="Example String" class="Str"(error in=w280, "Text.Justify"=w277) -> (error out=w279:errorcluster)  [unwired: 1 in, 1 out]
            n154 = property on="Example Button" class="Bool (严格)"(error in=w279, "BoolText.Justify"=w277) -> (error out=w278:errorcluster)  [unwired: 1 in, 1 out]
          }
          event "Font": Value Change {
            # "Error"
            # "Display State"
            n155 = event-data() -> ("NewVal"=w290:u16)  [unwired: 1 in]
            n156 = property on="Font" class="Ring (严格)"() -> ("Strings []"=w289:string[])  [unwired: 2 in, 2 out]
            n157 = To Long Integer(number=w290) -> (32bit integer=w288:i32)
            n158 = Index Array(array=w289, index=w288) -> (element=w284:string)
            n159 = Bundle By Name(cluster=w292, "Font.Font Name"=w284) -> (w291:T1)
            n160 = property on="Example String" class="Str"(error in=w287, "Text.FontName"=w284) -> (error out=w286:errorcluster)  [unwired: 1 in, 1 out]
            n161 = property on="Example Button" class="Bool (严格)"(error in=w286, "BoolText.FontName"=w284) -> (error out=w285:errorcluster)  [unwired: 1 in, 1 out]
          }
        }
      }
    }
    frame #2 {
      # "Check to see if there are any changes to the State data and set Change to true if there is.  The output will inform whether there has been a state change."
      n162 = local read "Display State In"() -> (w318:T1)
      n163 = Not Equal?(x=w317, y=w318) -> (x != y?=w316:T8)
      n164 = Unbundle By Name(w316) -> ("On Text"=w315:bool, "Off Text"=w314:bool, "Current Color.On Color"=w313:bool, "Current Color.Text Color"=w312:bool, "Current Color.Off Color"=w311:bool, "Button Color.On Color"=w310:bool, "Button Color.Text Color"=w309:bool, "Button Color.Off Color"=w308:bool, "Hover Color.On Color"=w307:bool, "Hover Color.Text Color"=w306:bool, "Hover Color.Off Color"=w305:bool, "Show Boolean Text"=w304:bool, "Multiple Strings"=w301:bool, "Font.Font Name"=w300:bool, "Font.Size"=w299:bool, "Font.Bold"=w298:bool, "Font.Italic"=w297:bool, "Font.Underline"=w296:bool, "Font.Strikeout"=w295:bool, "Font.Alignment"=w294:bool)
      n165 = Compound Arithmetic op=OR(w315, w314, w313, w312, w311, w310, w309, w308, w307, w306, w305, w304, w301, w300, w299, w298, w297, w296, w295, w294) -> (→"Change":bool)
      "Display State Out" <- w317
      "Error Out" <- w302
    }
  }
